vi "QueryServer_GetRequest_Register.vi"(0 "gRPCid":T1, 3 "error in (no error)":errorcluster) -> (7 "gRPCid out":T1, 9 "eventname":string, 10 "error out":errorcluster)   [LabVIEW 2019, in "labview-grpc-query-server.lvlib"]
uses:
  labview-grpc-query-server.lvlib
  VIs/grpcId.ctl
  QueryServer_RegisterRequest.ctl
  build/Debug/labview_grpc_server.dll
  VIs/gprc-support.lvlib
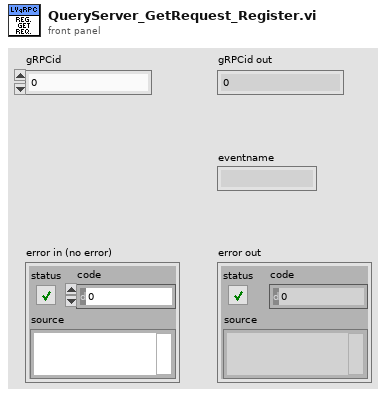
[diagram p1: front panel]
types:
  T1 = typedef "gprc-support.lvlib/grpcId.ctl" = u64
  T2 = typedef "labview-grpc-query-server.lvlib/QueryServer_RegisterRequest.ctl" = cluster{"eventname":string}
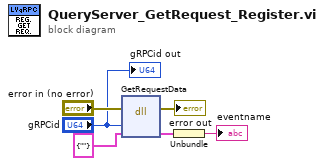
[diagram p0: block diagram]
diagram:
  n1 = dll-call lib="C:/dev/labview-grpc-server/build/Debug/labview_grpc_server.dll" fn="GetRequestData"(error in="error in (no error)", "id"="gRPCid", "data"=T2 {"eventname"=""} ("RegistrationRequest")) -> (error out=→"error out":errorcluster, "data"=w2:T2)  [unwired: 4 in, 1 out]
  n2 = Unbundle(w2) -> ("eventname"=→"eventname":string)
  "gRPCid out" <- "gRPCid"
